vi "Set Package Version.vi"(8 "error in (no error)":errorcluster, 9 "version":string, 10 "package name":string, 11 "NI Package Builder solution (.pbs)":path) -> (0 "error out":errorcluster, 2 "package name out":string, 3 "NI Package Builder solution out":path)   [LabVIEW 2017, in "NIPB Solution API.lvlib"]
doc: "Sets the version of the specified package in the specified NI Package Builder solution (.pbs).\n\nIf the <b>package name</b> input is unwired, this VI will perform this operation on the first package in the NI Package Builder solution and output the corresponding package name in the <b>package name out</b> output."
uses:
  NIPB Solution API.lvlib
  <vilib>/xml/NI_XML.lvlib
  <resource>/objmgr/DOMUserDefRef.rc
  <vilib>/xml/Load XML String.vi
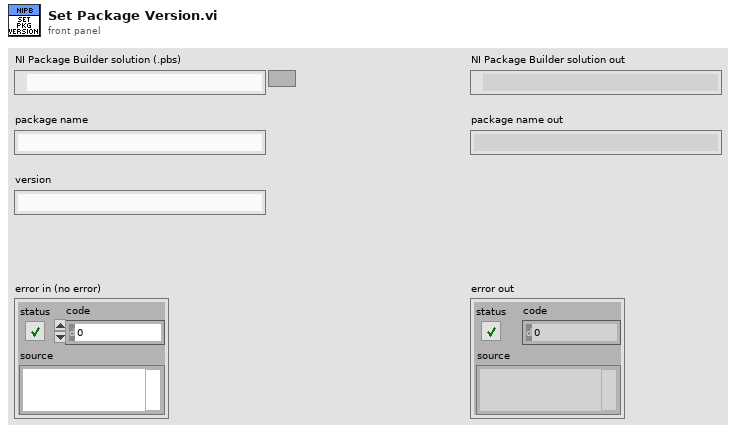
[diagram p1: front panel]
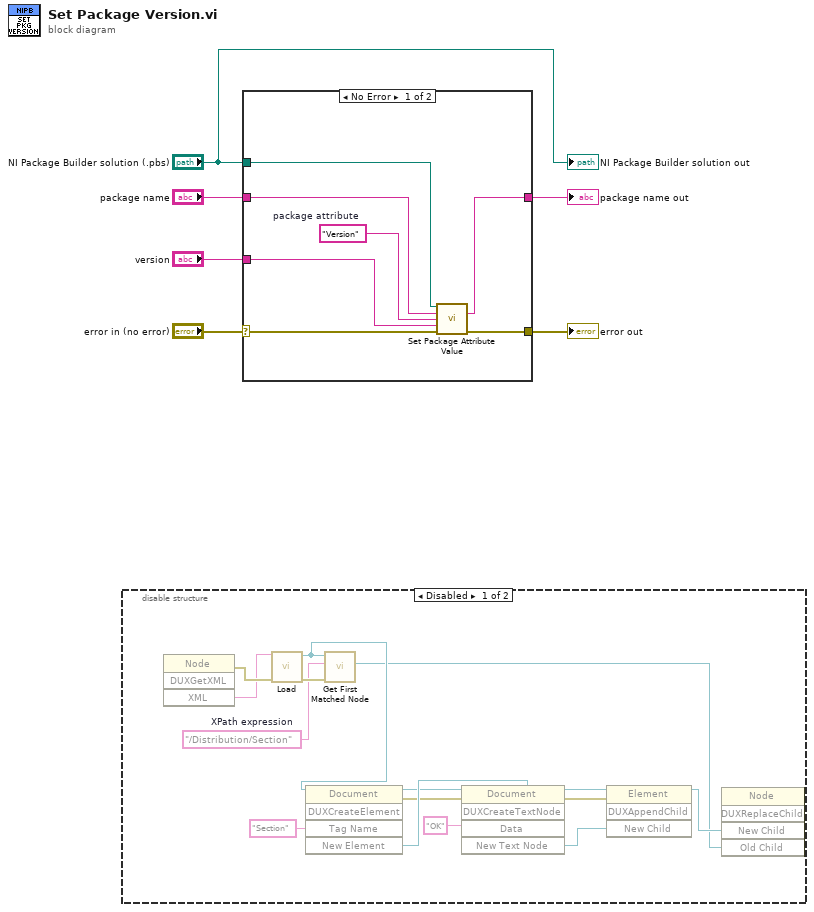
[diagram p0: block diagram]
diagram:
  n1 = disable-structure shown="Disabled" {
    frame Disabled {
      w11 = "/Distribution/Section"  # XPath expression
      n2 = invoke class="Node" method="DUXGetXML"() -> (reference=w7:refnum<k20>, error out=w13:errorcluster, "XML"=w12:string)  [unwired: 3 in, 2 out]
      n3 = call-poly <vilib>:"Load.vi"("XML string"=w12, "error in (no error)"=w13) -> ("DOM document out"=w10:refnum<k20>, "error out"=w14:errorcluster)  [unwired: 11 in, 1 out]
      n4 = invoke class="Document" method="DUXCreateElement"(reference=w10, "Tag Name"="Section") -> (reference out=w18:refnum<k20>, error out=w17:errorcluster, "New Element"=w20:refnum<k20>)  [unwired: 3 in, 2 out]
      n5 = call <vilib>:"Get First Matched Node.vi"("error in (no error)"=w14, "XPath expression"=w11, "node in"=w10) -> ("node result"=w9:refnum<k20>)  [unwired: 6 in, 2 out]
      n6 = invoke class="Document" method="DUXCreateTextNode"(reference=w18, error in=w17, "Data"="OK") -> (error out=w19:errorcluster, "New Text Node"=w21:refnum<k20>)  [unwired: 2 in, 3 out]
      n7 = invoke class="Element" method="DUXAppendChild"(reference=w20, error in=w19, "New Child"=w21) -> (reference out=w22:refnum<k20>)  [unwired: 1 in, 3 out]
      n8 = invoke class="Node" method="DUXReplaceChild"("New Child"=w22, "Old Child"=w9) -> (reference=w8:refnum<k20>)  [unwired: 2 in, 5 out]
    }
    frame Enabled {
    }
  }
  n9 = case shown="No Error" "error in (no error)" {
    selector: "error in (no error)" -> [w29 w31]
    tunnel: [w25 w31] -> w5
    tunnel: "NI Package Builder solution (.pbs)" -> [w27 _]
    tunnel: "package name" -> [w26 w30]
    tunnel: "version" -> [w28 _]
    tunnel: [w23 w30] -> w1
    frame No Error {
      w24 = "Version"  # package attribute
      n10 = call "Set Package Attribute Value.vi"("NI Package Builder solution (.pbs)"=w27, "package name"=w26, "package attribute"=w24, "value"=w28, "error in (no error)"=w29) -> ("package name out"=w23:string, "error out"=w25:errorcluster)  [unwired: 8 in, 1 out]
    }
    frame Error {
    }
  }
  "error out" <- w5
  "package name out" <- w1
  "NI Package Builder solution out" <- "NI Package Builder solution (.pbs)"
